vi "10_Alarms_u_1.vi"() -> ()   [LabVIEW 2011]
uses:
  <vilib>/Utility/miscctls.llb/LVPositionTypeDef.ctl
  Globals/Global VI.vi
  Globals/Global Alarm.vi
panel:
  in  "Up Button 2":bool
  in  "Down Button 2":bool
  in  "Down Button":bool
  in  "Up Button":bool
  in  "Alarm History":i32(listbox)
  in  "Active Alarms":i32(listbox)
  # "Alarms"
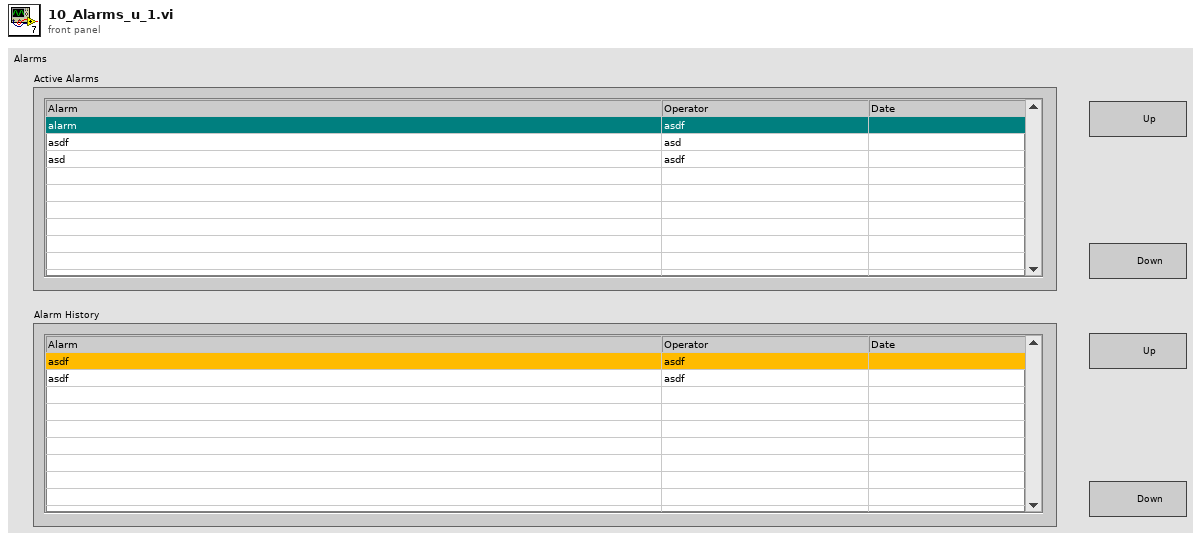
[diagram p1: front panel]
types:
  T1 = typedef "LVPositionTypeDef.ctl" = cluster{"Left":i32, "Top":i32}
  T2 = typedef "LVAllMonitorsDisplayTypeDef.ctl" = cluster{"Bounds":cluster{"Left":i16, "Top":i16, "Right":i16, "Bottom":i16}, "Depth":i16}[]
  T3 = cluster{"Bounds":cluster{"Left":i16, "Top":i16, "Right":i16, "Bottom":i16}, "Depth":i16}
  T4 = typedef "LVRowAndColumnUnsignedTypeDef.ctl" = cluster{"Row":u32, "Column":u32}
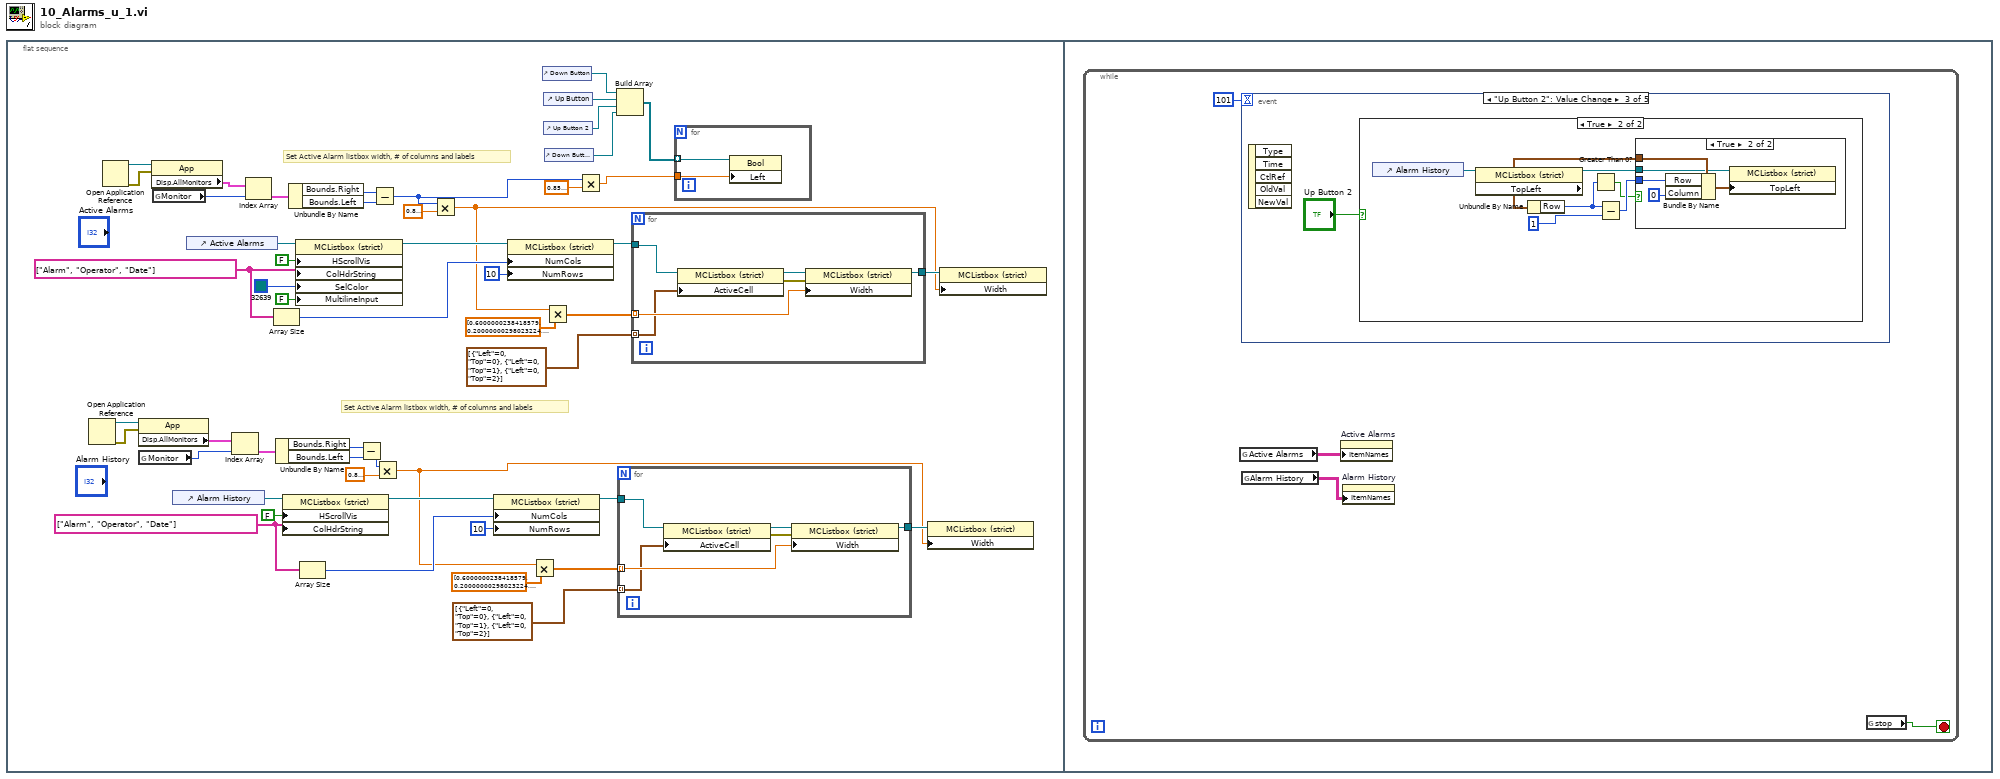
[diagram p0: block diagram]
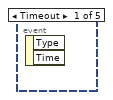
[diagram p2: hidden frame]
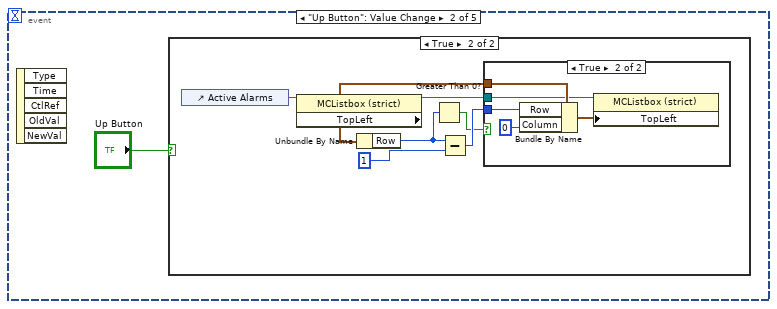
[diagram p3: hidden frame]
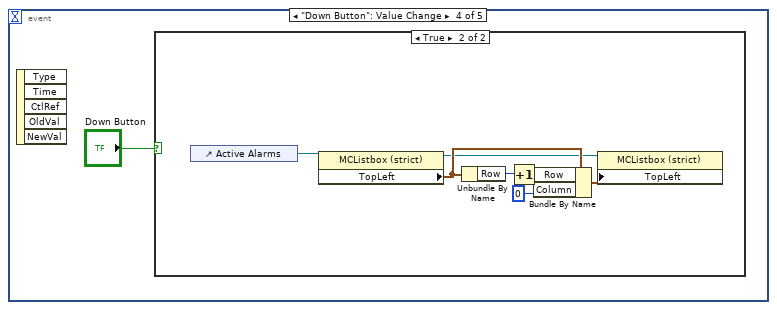
[diagram p8: hidden frame]
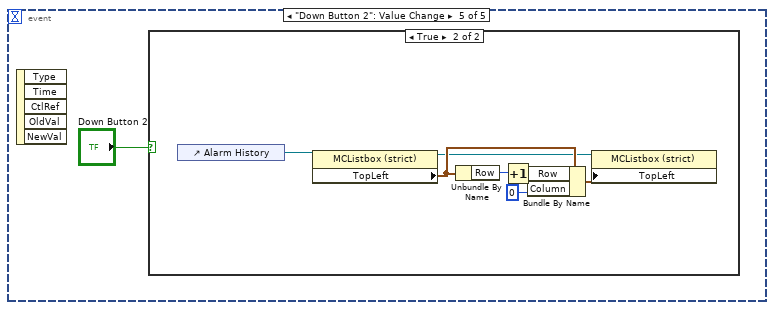
[diagram p10: hidden frame]
diagram:
  n1 = flat-sequence {
    frame #0 {
      w26 = string[] ["Alarm", "Operator", "Date"] ("Column Header Strings[]")
      w43 = string[] ["Alarm", "Operator", "Date"] ("Column Header Strings[]")
      # "Set Active Alarm listbox width, # of columns and labels"
      # "Set Active Alarm listbox width, # of columns and labels"
      n2 = Open Application Reference() -> (0:w17:errorcluster, 3:w18:refnum<vi>)  [unwired: 4 in]
      n3 = Open Application Reference() -> (0:w50:errorcluster, 3:w49:refnum<vi>)  [unwired: 4 in]
      n4 = property class="App"(reference=w18, error in=w17) -> ("Disp.AllMonitors"=w19:T2)  [unwired: 2 out]
      n5 = global read "Global VI.vi" "Monitor"() -> (w21:u16)
      n6 = property class="App"(reference=w49, error in=w50) -> ("Disp.AllMonitors"=w48:T2)  [unwired: 2 out]
      n7 = global read "Global VI.vi" "Monitor"() -> (w46:u16)
      n8 = control-ref of="Alarm History"() -> (w27:refnum<vi>)
      n9 = control-ref of="Active Alarms"() -> (w42:refnum<vi>)
      n10 = Index Array(array=w19, index=w21) -> (element=w20:T3)
      n11 = Index Array(array=w48, index=w46) -> (element=w47:T3)
      n12 = Array Size(array=w43) -> (size(s)=w38:i32)
      n13 = Unbundle By Name(w20) -> ("Bounds.Right"=w23:i16, "Bounds.Left"=w22:i16)
      n14 = property class="MCListbox (strict)"(reference=w27, "HScrollVis"=FALSE ("Visible Items:Horizontal Scrollbar Visible"), "ColHdrString"=w26) -> (reference out=w33:refnum<vi>)  [unwired: 1 in, 1 out]
      n15 = Unbundle By Name(w47) -> ("Bounds.Right"=w45:i16, "Bounds.Left"=w7:i16)
      n16 = property class="MCListbox (strict)"(reference=w42, "HScrollVis"=FALSE ("Visible Items:Horizontal Scrollbar Visible"), "ColHdrString"=w43, "SelColor"=u32 32639, "MultilineInput"=FALSE ("Multiple Line Input")) -> (reference out=w36:refnum<vi>)  [unwired: 1 in, 1 out]
      n17 = Array Size(array=w26) -> (size(s)=w31:i32)
      n18 = Subtract(x=w23, y=w22) -> (x-y=w24:i16)
      n19 = Subtract(x=w45, y=w7) -> (x-y=w8:i16)
      n20 = Multiply(x=w24, y=sgl 0.8) -> (x*y=w12:sgl)
      n21 = Multiply(x=w8, y=sgl 0.8) -> (x*y=w14:sgl)
      n22 = property class="MCListbox (strict)"(reference=w33, "NumCols"=w31, "NumRows"=u32 10 ("Number of Rows")) -> (reference out=w32:refnum<vi>)  [unwired: 1 in, 1 out]
      n23 = property class="MCListbox (strict)"(reference=w36, "NumCols"=w38, "NumRows"=u32 10 ("Number of Rows")) -> (reference out=w37:refnum<vi>)  [unwired: 1 in, 1 out]
      n24 = Multiply(x=w12, y=sgl[] [0.6, 0.2, 0.2]) -> (x*y=w30:sgl[])
      n25 = control-ref of="Down Button"() -> (w6:refnum<vi>)
      n26 = control-ref of="Up Button"() -> (w5:refnum<vi>)
      n27 = control-ref of="Up Button 2"() -> (w3:refnum<vi>)
      n28 = control-ref of="Down Button 2"() -> (w2:refnum<vi>)
      n29 = Multiply(x=w14, y=sgl[] [0.6, 0.2, 0.2]) -> (x*y=w39:sgl[])
      n30 = Multiply(x=w8, y=sgl 0.85) -> (x*y=w1:sgl)
      n31 = Build Array(w6, w5, w3, w2) -> (w4:refnum<vi>[])
      n32 = for {
        tunnel: w32 -> [w55]
        tunnel: T1[] [{"Left"=0, "Top"=0}, {"Left"=0, "Top"=1}, {"Left"=0, "Top"=2}] -> [w56] mode=indexing
        tunnel: w30 -> [w57] mode=indexing
        tunnel: [w54] -> w13
        n33 = property class="MCListbox (strict)"(reference=w55, "ActiveCell"=w56) -> (reference out=w59:refnum<vi>, error out=w58:errorcluster)  [unwired: 1 in]
        n34 = property class="MCListbox (strict)"(reference=w59, error in=w58, "Width"=w57) -> (reference out=w54:refnum<vi>)  [unwired: 1 out]
      }
      n35 = for {
        tunnel: w37 -> [w61]
        tunnel: T1[] [{"Left"=0, "Top"=0}, {"Left"=0, "Top"=1}, {"Left"=0, "Top"=2}] -> [w62] mode=indexing
        tunnel: w39 -> [w63] mode=indexing
        tunnel: [w60] -> w15
        n36 = property class="MCListbox (strict)"(reference=w61, "ActiveCell"=w62) -> (reference out=w65:refnum<vi>, error out=w64:errorcluster)  [unwired: 1 in]
        n37 = property class="MCListbox (strict)"(reference=w65, error in=w64, "Width"=w63) -> (reference out=w60:refnum<vi>)  [unwired: 1 out]
      }
      n38 = for {
        tunnel: w1 -> [w53]
        tunnel: w4 -> [w52] mode=indexing
        n39 = property class="Bool"(reference=w52, "Left"=w53) -> ()  [unwired: 1 in, 2 out]
      }
      n40 = property class="MCListbox (strict)"(reference=w13, "Width"=w12) -> ()  [unwired: 1 in, 2 out]
      n41 = property class="MCListbox (strict)"(reference=w15, "Width"=w14) -> ()  [unwired: 1 in, 2 out]
    }
    frame #1 {
      n42 = while {
        stop <- w69 stop-if-true
        n43 = global read "Global Alarm.vi" "Active Alarms"() -> (w67:string[][])
        n44 = event shown="[2] \"Up Button 2\": Value Change" {
          selector: _ -> [_ _ _ _ _]
          dyn-events: _ -> [_ _ _ _ _]
          timeout: 101 -> [_ _ _ _ _]
          event Timeout {
            n45 = event-data() -> ()  [unwired: 1 in, 2 out]
          }
          event "Up Button": Value Change {
            n46 = event-data() -> ()  [unwired: 1 in, 5 out]
            n47 = case shown="True" "Up Button" {
              frame False {
              }
              frame True {
                n48 = control-ref of="Active Alarms"() -> (w77:refnum<vi>)
                n49 = property class="MCListbox (strict)"(reference=w77) -> (reference out=w75:refnum<vi>, "TopLeft"=w76:T4)  [unwired: 1 in, 1 out]
                n50 = Unbundle By Name(w76) -> ("Row"=w71:u32)
                n51 = Greater Than 0?(x=w71) -> (x > 0?=w72:bool)
                n52 = Subtract(x=w71, y=u32 1) -> (x-y=w73:u32)
                n53 = case shown="True" w72 {
                  tunnel: w76 -> [_ w81]
                  tunnel: w75 -> [_ w80]
                  tunnel: w73 -> [_ w78]
                  frame False {
                  }
                  frame True {
                    n54 = Bundle By Name(cluster=w81, "Row"=w78, "Column"=u32 0) -> (w82:T4)
                    n55 = property class="MCListbox (strict)"(reference=w80, "TopLeft"=w82) -> ()  [unwired: 1 in, 2 out]
                  }
                }
              }
            }
          }
          event "Up Button 2": Value Change {
            n56 = event-data() -> ()  [unwired: 1 in, 5 out]
            n57 = case shown="True" "Up Button 2" {
              frame False {
              }
              frame True {
                n58 = control-ref of="Alarm History"() -> (w84:refnum<vi>)
                n59 = property class="MCListbox (strict)"(reference=w84) -> (reference out=w89:refnum<vi>, "TopLeft"=w90:T4)  [unwired: 1 in, 1 out]
                n60 = Unbundle By Name(w90) -> ("Row"=w85:u32)
                n61 = Greater Than 0?(x=w85) -> (x > 0?=w86:bool)
                n62 = Subtract(x=w85, y=u32 1) -> (x-y=w87:u32)
                n63 = case shown="True" w86 {
                  tunnel: w90 -> [_ w94]
                  tunnel: w89 -> [_ w93]
                  tunnel: w87 -> [_ w91]
                  frame False {
                  }
                  frame True {
                    n64 = Bundle By Name(cluster=w94, "Row"=w91, "Column"=u32 0) -> (w95:T4)
                    n65 = property class="MCListbox (strict)"(reference=w93, "TopLeft"=w95) -> ()  [unwired: 1 in, 2 out]
                  }
                }
              }
            }
          }
          event "Down Button": Value Change {
            n66 = event-data() -> ()  [unwired: 1 in, 5 out]
            n67 = case shown="True" "Down Button" {
              frame False {
              }
              frame True {
                n68 = control-ref of="Active Alarms"() -> (w103:refnum<vi>)
                n69 = property class="MCListbox (strict)"(reference=w103) -> (reference out=w98:refnum<vi>, "TopLeft"=w100:T4)  [unwired: 1 in, 1 out]
                n70 = Unbundle By Name(w100) -> ("Row"=w102:u32)
                n71 = Increment(x=w102) -> (x+1=w99:u32)
                n72 = Bundle By Name(cluster=w100, "Row"=w99, "Column"=0) -> (w101:T4)
                n73 = property class="MCListbox (strict)"(reference=w98, "TopLeft"=w101) -> ()  [unwired: 1 in, 2 out]
              }
            }
          }
          event "Down Button 2": Value Change {
            n74 = event-data() -> ()  [unwired: 1 in, 5 out]
            n75 = case shown="True" "Down Button 2" {
              frame False {
              }
              frame True {
                n76 = control-ref of="Alarm History"() -> (w105:refnum<vi>)
                n77 = property class="MCListbox (strict)"(reference=w105) -> (reference out=w107:refnum<vi>, "TopLeft"=w109:T4)  [unwired: 1 in, 1 out]
                n78 = Unbundle By Name(w109) -> ("Row"=w111:u32)
                n79 = Increment(x=w111) -> (x+1=w108:u32)
                n80 = Bundle By Name(cluster=w109, "Row"=w108, "Column"=0) -> (w110:T4)
                n81 = property class="MCListbox (strict)"(reference=w107, "TopLeft"=w110) -> ()  [unwired: 1 in, 2 out]
              }
            }
          }
        }
        n82 = global read "Global Alarm.vi" "Alarm History"() -> (w66:string[][])
        n83 = property on="Active Alarms" class="MCListbox (strict)"("ItemNames"=w67) -> ()  [unwired: 2 in, 2 out]
        n84 = property on="Alarm History" class="MCListbox (strict)"("ItemNames"=w66) -> ()  [unwired: 2 in, 2 out]
        n85 = global read "Global VI.vi" "stop"() -> (w69:bool)
      }
    }
  }
